vi "insert and parse tests.vi"() -> ()   [LabVIEW 2015]
uses:
  API/JSON Document Class/json insert/poly instances/json Insert Boolean - string path.vi
  API/JSON Document Class/json parse/poly instances/json Parse Boolean - string path.vi
  API/JSON Document Class/json insert/poly instances/json Insert Double - string path.vi
  API/JSON Document Class/json parse/poly instances/json Parse Double - string path.vi
  API/JSON Document Class/json insert/poly instances/json Insert Float - string path.vi
  API/JSON Document Class/json parse/poly instances/json Parse Float - string path.vi
  API/JSON Document Class/json insert/poly instances/json Insert U64 - string path.vi
  API/JSON Document Class/json parse/poly instances/json Parse U64 - string path.vi
  API/JSON Document Class/json insert/poly instances/json Insert U32 - string path.vi
  API/JSON Document Class/json parse/poly instances/json Parse U32 - string path.vi
  API/JSON Document Class/json insert/poly instances/json Insert I32 - string path.vi
  API/JSON Document Class/json parse/poly instances/json Parse I32 - string path.vi
  API/JSON Document Class/json insert/poly instances/json Insert I64 - string path.vi
  API/JSON Document Class/json parse/poly instances/json Parse I64 - string path.vi
  API/JSON Document Class/json insert/poly instances/json Insert String - string path.vi
  API/JSON Document Class/json parse/poly instances/json Parse String - string path.vi
  API/JSON Document Class/json insert/poly instances/json Insert Boolean Array - string path.vi
  API/JSON Document Class/json parse/poly instances/json Parse Boolean Array - string path.vi
  API/JSON Document Class/json to string/json To Pretty String - string path.vi
  API/JSON Document Class/JSON Document.lvclass
panel:
  out "Member Names":string[](array[string])
  out "value 4":bool[](array[boolean])
  out "json string":string
  out "replaced? 8":bool
  out "string":string
  out "found? 8":bool
  out "value 2":i64
  out "found? 7":bool
  out "replaced? 7":bool
  out "value":i32
  out "found? 6":bool
  out "replaced? 6":bool
  out "u32":u32
  out "found? 5":bool
  out "replaced? 5":bool
  out "u64":u64
  out "found? 4":bool
  out "replaced? 4":bool
  out "single":sgl
  out "found? 3":bool
  out "replaced? 3":bool
  out "found? 2":bool
  out "double":dbl
  out "replaced? 2":bool
  out "found?":bool
  out "boolean":bool
  out "replaced?":bool
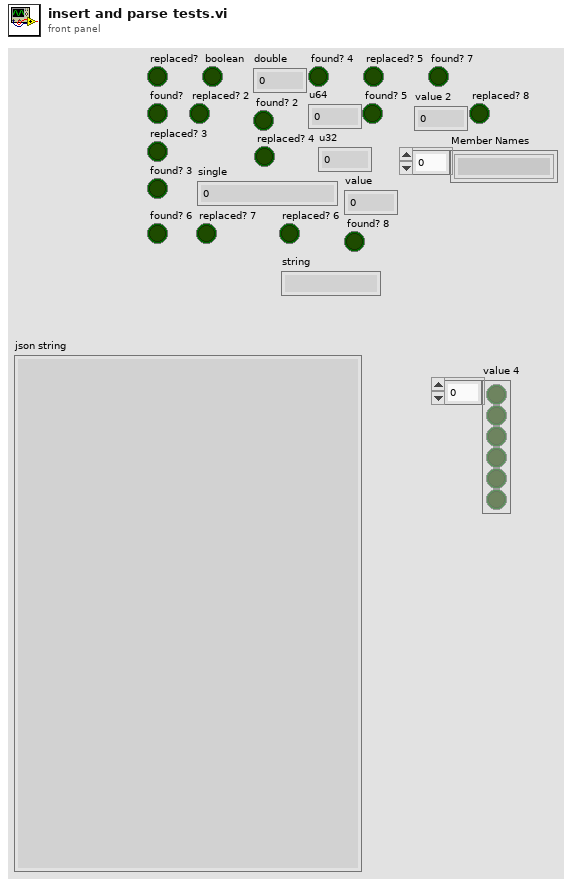
[diagram p1: front panel]
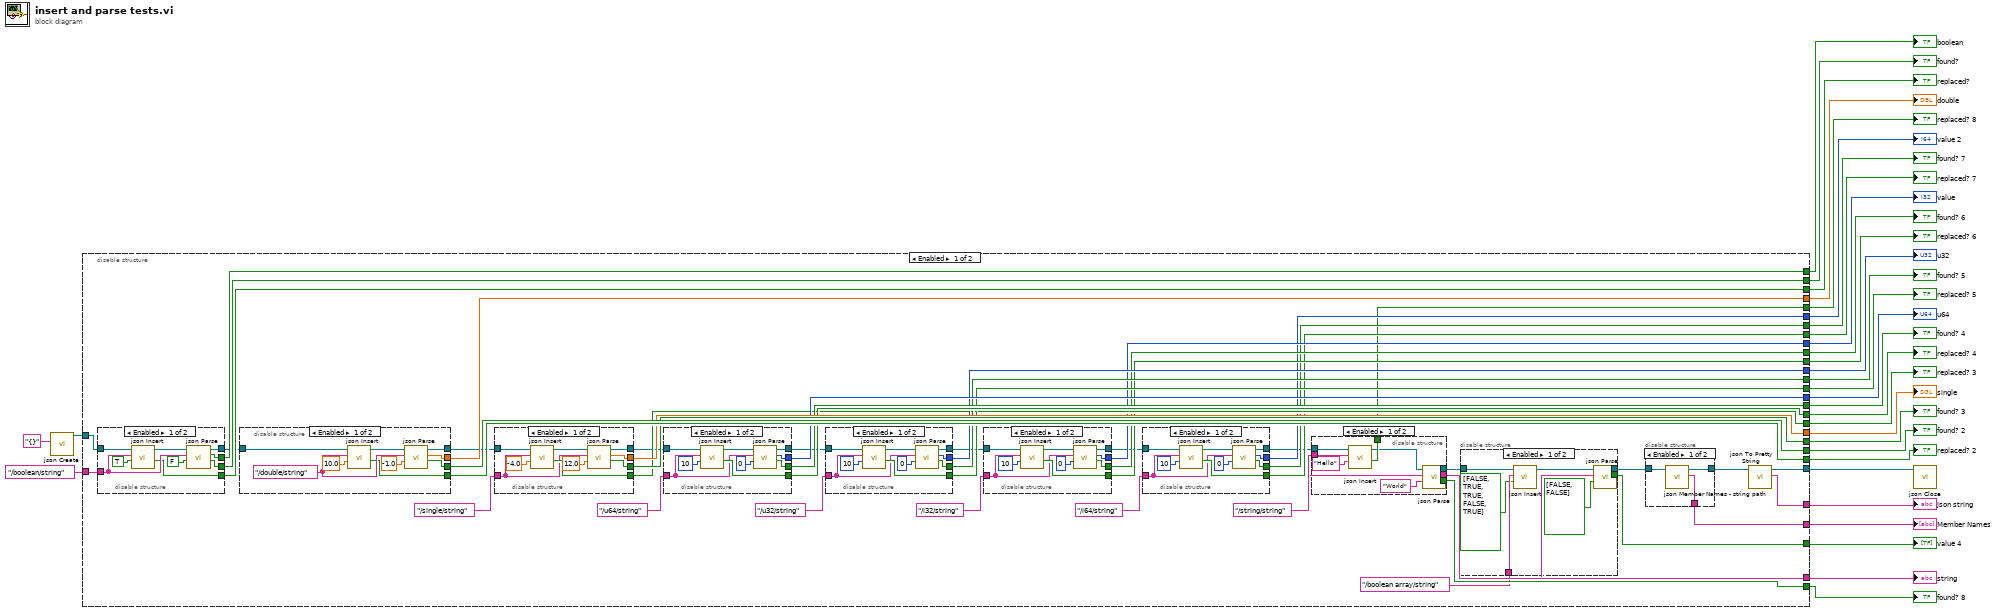
[diagram p0: block diagram]
diagram:
  n1 = call "json Create.vi"("JSON String"="{}") -> ("JSON Document out"=w31:refnum<class "JSON Document.lvclass">)  [unwired: 9 in, 1 out]
  n2 = disable-structure shown="Enabled" {
    disable-tunnel: w31 -> [w78 w171]
    disable-tunnel: "/boolean/string" ("path") -> [w77 _]
    disable-tunnel: [w76 _] -> w29
    disable-tunnel: [w75 _] -> w28
    disable-tunnel: [w74 _] -> w27
    disable-tunnel: [w72 _] -> w25
    disable-tunnel: [w71 _] -> w24
    disable-tunnel: [w70 _] -> w23
    disable-tunnel: [w69 _] -> w22
    disable-tunnel: [w68 _] -> w21
    disable-tunnel: [w67 _] -> w20
    disable-tunnel: [w66 _] -> w19
    disable-tunnel: [w65 _] -> w18
    disable-tunnel: [w64 _] -> w17
    disable-tunnel: [w63 _] -> w16
    disable-tunnel: [w62 _] -> w15
    disable-tunnel: [w61 _] -> w14
    disable-tunnel: [w60 _] -> w13
    disable-tunnel: [w59 _] -> w12
    disable-tunnel: [w58 _] -> w11
    disable-tunnel: [w57 _] -> w10
    disable-tunnel: [w56 _] -> w9
    disable-tunnel: [w55 _] -> w8
    disable-tunnel: [w54 _] -> w7
    disable-tunnel: [w53 _] -> w6
    disable-tunnel: [w52 _] -> w5
    disable-tunnel: [w51 w171] -> w4
    disable-tunnel: [w50 _] -> w3
    disable-tunnel: [w49 _] -> w2
    disable-tunnel: [w48 _] -> w1
    frame Enabled {
      n3 = disable-structure shown="Enabled" {
        disable-tunnel: w78 -> [w169 w170]
        disable-tunnel: w77 -> [w166 _]
        disable-tunnel: [w164 _] -> w76
        disable-tunnel: [w163 _] -> w75
        disable-tunnel: [w162 _] -> w74
        disable-tunnel: [w161 w170] -> w73
        frame Enabled {
          n4 = call-poly "json Insert.vi"("anything"=TRUE, "path"=w166, "JSON Document in"=w169) -> ("replaced?"=w164:bool, "JSON Document out"=w167:refnum<class "JSON Document.lvclass">)  [unwired: 6 in, 1 out]
          n5 = call-poly "json Parse.vi"("default"=FALSE, "path"=w166, "JSON Document in"=w167) -> ("defaulted?"=w162:bool, "value"=w163:bool, "JSON Document out"=w161:refnum<class "JSON Document.lvclass">)  [unwired: 5 in, 1 out]
        }
        frame Disabled {
        }
      }
      n6 = disable-structure shown="Enabled" {
        disable-tunnel: w73 -> [w159 w160]
        disable-tunnel: [w157 _] -> w72
        disable-tunnel: [w156 _] -> w71
        disable-tunnel: [w155 _] -> w70
        disable-tunnel: [w153 w160] -> w47
        frame Enabled {
          w158 = "/double/string" ("path")
          n7 = call-poly "json Insert.vi"("anything"=10.0, "path"=w158, "JSON Document in"=w159) -> ("replaced?"=w157:bool, "JSON Document out"=w154:refnum<class "JSON Document.lvclass">)  [unwired: 6 in, 1 out]
          n8 = call-poly "json Parse.vi"("default"=-1.0, "path"=w158, "JSON Document in"=w154) -> ("defaulted?"=w155:bool, "value"=w156:dbl, "JSON Document out"=w153:refnum<class "JSON Document.lvclass">)  [unwired: 5 in, 1 out]
        }
        frame Disabled {
        }
      }
      n9 = disable-structure shown="Enabled" {
        disable-tunnel: [w149 _] -> w69
        disable-tunnel: [w148 _] -> w68
        disable-tunnel: [w147 _] -> w61
        disable-tunnel: w47 -> [w146 w150]
        disable-tunnel: [w145 w150] -> w46
        disable-tunnel: "/single/string" ("path") -> [w143 _]
        frame Enabled {
          n10 = call-poly "json Insert.vi"("anything"=sgl -4.0, "path"=w143, "JSON Document in"=w146) -> ("replaced?"=w147:bool, "JSON Document out"=w141:refnum<class "JSON Document.lvclass">)  [unwired: 6 in, 1 out]
          n11 = call-poly "json Parse.vi"("default"=sgl 12.0, "path"=w143, "JSON Document in"=w141) -> ("defaulted?"=w149:bool, "value"=w148:sgl, "JSON Document out"=w145:refnum<class "JSON Document.lvclass">)  [unwired: 5 in, 1 out]
        }
        frame Disabled {
        }
      }
      n12 = disable-structure shown="Enabled" {
        disable-tunnel: [w139 _] -> w67
        disable-tunnel: [w138 _] -> w66
        disable-tunnel: [w137 _] -> w65
        disable-tunnel: w46 -> [w136 w140]
        disable-tunnel: [w134 w140] -> w45
        disable-tunnel: "/u64/string" ("path") -> [w133 _]
        frame Enabled {
          n13 = call-poly "json Insert.vi"("anything"=u64 10, "path"=w133, "JSON Document in"=w136) -> ("replaced?"=w139:bool, "JSON Document out"=w135:refnum<class "JSON Document.lvclass">)  [unwired: 6 in, 1 out]
          n14 = call-poly "json Parse.vi"("default"=u64 0, "path"=w133, "JSON Document in"=w135) -> ("defaulted?"=w138:bool, "value"=w137:u64, "JSON Document out"=w134:refnum<class "JSON Document.lvclass">)  [unwired: 5 in, 1 out]
        }
        frame Disabled {
        }
      }
      n15 = disable-structure shown="Enabled" {
        disable-tunnel: [w129 _] -> w64
        disable-tunnel: [w128 _] -> w63
        disable-tunnel: [w127 _] -> w62
        disable-tunnel: w45 -> [w126 w130]
        disable-tunnel: "/u32/string" ("path") -> [w122 _]
        disable-tunnel: [w121 w130] -> w40
        frame Enabled {
          n16 = call-poly "json Insert.vi"("anything"=u32 10, "path"=w122, "JSON Document in"=w126) -> ("replaced?"=w129:bool, "JSON Document out"=w125:refnum<class "JSON Document.lvclass">)  [unwired: 6 in, 1 out]
          n17 = call-poly "json Parse.vi"("default"=u32 0, "path"=w122, "JSON Document in"=w125) -> ("defaulted?"=w128:bool, "value"=w127:u32, "JSON Document out"=w121:refnum<class "JSON Document.lvclass">)  [unwired: 5 in, 1 out]
        }
        frame Disabled {
        }
      }
      n18 = disable-structure shown="Enabled" {
        disable-tunnel: [w119 _] -> w60
        disable-tunnel: [w118 _] -> w59
        disable-tunnel: [w117 _] -> w58
        disable-tunnel: "/i32/string" ("path") -> [w116 _]
        disable-tunnel: w40 -> [w112 w120]
        disable-tunnel: [w111 w120] -> w38
        frame Enabled {
          n19 = call-poly "json Insert.vi"("anything"=10, "path"=w116, "JSON Document in"=w112) -> ("replaced?"=w119:bool, "JSON Document out"=w113:refnum<class "JSON Document.lvclass">)  [unwired: 6 in, 1 out]
          n20 = call-poly "json Parse.vi"("default"=0, "path"=w116, "JSON Document in"=w113) -> ("defaulted?"=w118:bool, "value"=w117:i32, "JSON Document out"=w111:refnum<class "JSON Document.lvclass">)  [unwired: 5 in, 1 out]
        }
        frame Disabled {
        }
      }
      n21 = disable-structure shown="Enabled" {
        disable-tunnel: [w109 _] -> w57
        disable-tunnel: [w108 _] -> w56
        disable-tunnel: [w107 _] -> w55
        disable-tunnel: "/i64/string" ("path") -> [w103 _]
        disable-tunnel: w38 -> [w102 w110]
        disable-tunnel: [w101 w110] -> w36
        frame Enabled {
          n22 = call-poly "json Insert.vi"("anything"=i64 10, "path"=w103, "JSON Document in"=w102) -> ("replaced?"=w109:bool, "JSON Document out"=w106:refnum<class "JSON Document.lvclass">)  [unwired: 6 in, 1 out]
          n23 = call-poly "json Parse.vi"("default"=i64 0, "path"=w103, "JSON Document in"=w106) -> ("defaulted?"=w108:bool, "value"=w107:i64, "JSON Document out"=w101:refnum<class "JSON Document.lvclass">)  [unwired: 5 in, 1 out]
        }
        frame Disabled {
        }
      }
      n24 = disable-structure shown="Enabled" {
        disable-tunnel: [w99 _] -> w54
        disable-tunnel: [w98 _] -> w53
        disable-tunnel: [w97 _] -> w52
        disable-tunnel: "/string/string" ("path") -> [w96 _]
        disable-tunnel: w36 -> [w94 w100]
        disable-tunnel: [w91 w100] -> w35
        frame Enabled {
          n25 = call-poly "json Insert.vi"("anything"="Hello" ("path"), "path"=w96, "JSON Document in"=w94) -> ("replaced?"=w97:bool, "JSON Document out"=w95:refnum<class "JSON Document.lvclass">)  [unwired: 6 in, 1 out]
          n26 = call-poly "json Parse.vi"("default"="World" ("path"), "path"=w96, "JSON Document in"=w95) -> ("defaulted?"=w99:bool, "value"=w98:string, "JSON Document out"=w91:refnum<class "JSON Document.lvclass">)  [unwired: 5 in, 1 out]
        }
        frame Disabled {
        }
      }
      n27 = disable-structure shown="Enabled" {
        disable-tunnel: [w89 _] -> w49
        disable-tunnel: w35 -> [w88 w90]
        disable-tunnel: [w87 w90] -> w34
        disable-tunnel: "/boolean array/string" ("path") -> [w84 _]
        frame Enabled {
          n28 = call-poly "json Insert.vi"("anything"=bool[] [FALSE, TRUE, TRUE, FALSE, TRUE], "path"=w84, "JSON Document in"=w88) -> ("JSON Document out"=w86:refnum<class "JSON Document.lvclass">)  [unwired: 6 in, 2 out]
          n29 = call-poly "json Parse.vi"("default"=bool[] [FALSE, FALSE], "path"=w84, "JSON Document in"=w86) -> ("value"=w89:bool[], "JSON Document out"=w87:refnum<class "JSON Document.lvclass">)  [unwired: 4 in, 3 out]
        }
        frame Disabled {
        }
      }
      n30 = disable-structure shown="Enabled" {
        disable-tunnel: [w81 _] -> w48
        disable-tunnel: w34 -> [w80 w82]
        disable-tunnel: [w79 w82] -> w33
        frame Enabled {
          n31 = call "json Member Names - string path.vi"("JSON Document in"=w80) -> ("Member Names"=w81:string[], "JSON Document out"=w79:refnum<class "JSON Document.lvclass">)  [unwired: 8 in, 1 out]
        }
        frame Disabled {
        }
      }
      n32 = call-poly "json To Pretty String.vi"("JSON Document in"=w33) -> ("json string"=w50:string, "JSON Document out"=w51:refnum<class "JSON Document.lvclass">)  [unwired: 8 in, 1 out]
    }
    frame Disabled {
    }
  }
  "replaced?" <- w29
  "boolean" <- w28
  "found?" <- w27
  "replaced? 2" <- w25
  "double" <- w24
  "found? 2" <- w23
  "replaced? 3" <- w14
  "found? 3" <- w22
  "single" <- w21
  "replaced? 4" <- w20
  "found? 4" <- w19
  "u64" <- w18
  "replaced? 5" <- w17
  "found? 5" <- w16
  "u32" <- w15
  "replaced? 6" <- w13
  "found? 6" <- w12
  "value" <- w11
  "replaced? 7" <- w10
  "found? 7" <- w9
  "value 2" <- w8
  "found? 8" <- w7
  "string" <- w6
  "replaced? 8" <- w5
  "json string" <- w3
  "value 4" <- w2
  "Member Names" <- w1
  n33 = call "json Close.vi"("JSON Document in"=w4) -> ()  [unwired: 10 in, 1 out]
